vi "Import Groups.vi"(8 "error in (no error)":errorcluster, 10 "Path":path, 11 "BluelinesRedlines in":refnum<class "BluelinesRedlines.lvclass">) -> (0 "error out":errorcluster, 3 "BluelinesRedlines out":refnum<class "BluelinesRedlines.lvclass">)   [LabVIEW 2023, in "VolatusGUIElements.lvlib" / "BluelinesRedlines.lvclass"]
uses:
  BluelinesRedlines.lvclass
  VolatusGUI/BluelinesRedlines Source/BLRL Type.ctl
  BluelinesRedlines.lvclass/BluelinesRedlines.ctl
  User BluelinesRedlines/User BluelinesRedlines.lvclass
  VolatusErrorUtilities/MultiErrors/MultiErrors.lvclass/MultiErrors.ctl
  lv-cdm/CDM-Config/Config-JSON/Config-JSON.lvclass
  lv-cdm/CDM-Config/Config Storage/Config Storage.lvclass
  lv-cdm/CDM-Config/Config Manager/Config Manager.lvclass
  lv-cdm/CDM-Config/Config Element/Config Element.lvclass
  VolatusGUI/BluelinesRedlines Source/BluelinesRedlines Source.lvclass
  VolatusErrorUtilities/MultiErrors/MultiErrors.lvclass
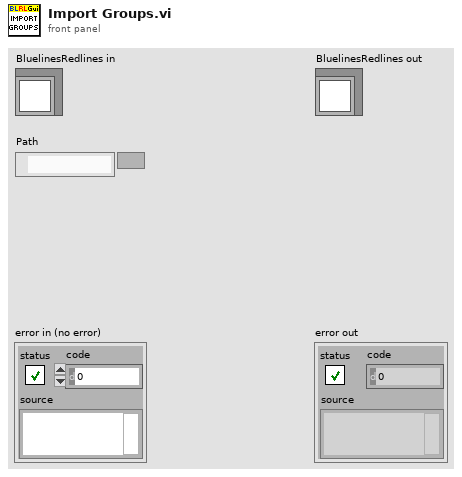
[diagram p1: front panel]
types:
  T1 = typedef "VolatusGUI.lvlib/BluelinesRedlines Source.lvclass/BLRL Type.ctl" = enum16{"Blueline", "Redline"}
  T2 = map{string, refnum<class "BluelinesRedlines Source.lvclass">}
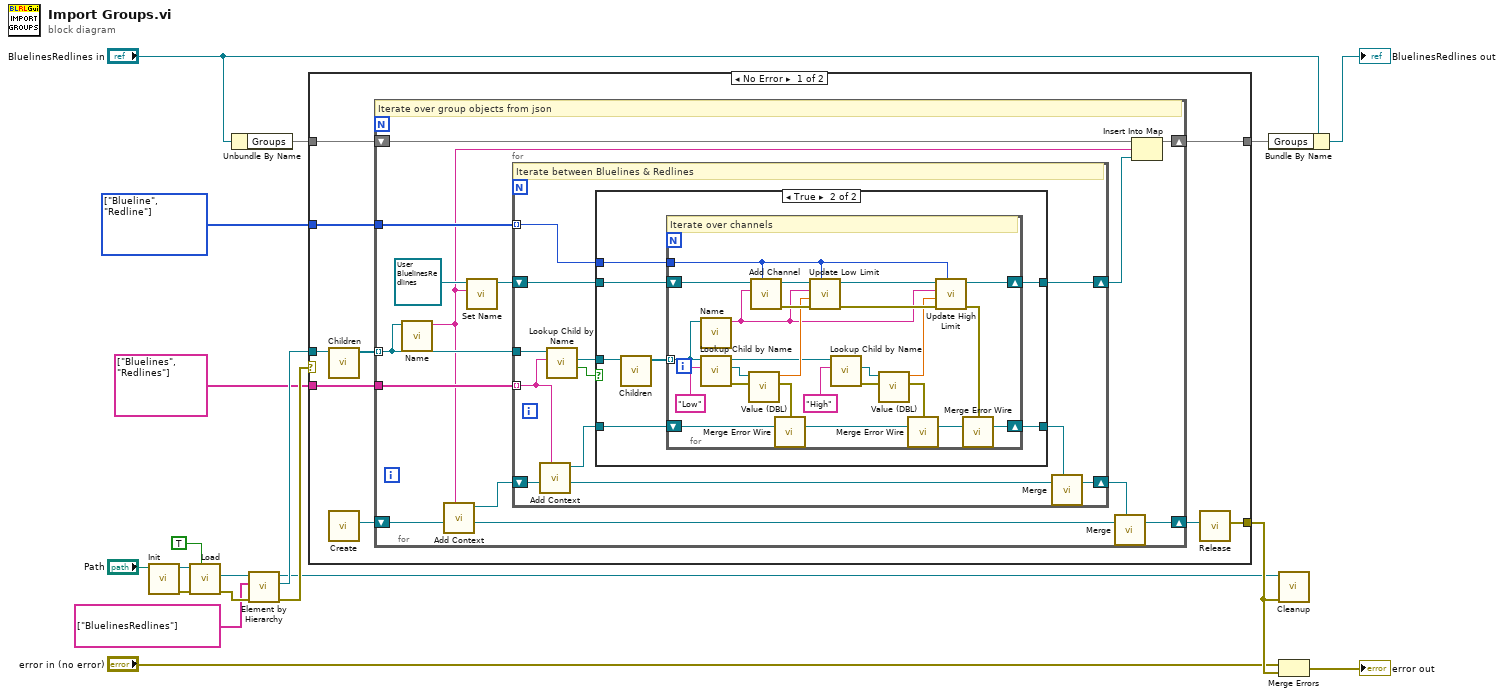
[diagram p0: block diagram]
diagram:
  w2 = T1[] [enum."Blueline", enum."Redline"] items=["Blueline", "Redline"]
  n1 = call "Init.vi"("Path"="Path") -> ("error out"=w15:errorcluster, "Config-JSON out"=w16:refnum<class "Config-JSON.lvclass">)  [unwired: 9 in]
  n2 = call "Load.vi"("Mutable (F)"=TRUE, "error in (no error)"=w15, "Config Storage in"=w16) -> ("error out"=w13:errorcluster, "Config"=w14:refnum<class "Config Manager.lvclass">)  [unwired: 6 in, 1 out]
  n3 = Unbundle By Name("BluelinesRedlines in") -> ("Groups"=w6:T2)
  n4 = call "Element by Hierarchy.vi"("error in (no error)"=w13, "Hierarchy"=string[] ["BluelinesRedlines"], "Config Manager in"=w14) -> ("error out"=w11:errorcluster, "Config Element"=w10:refnum<class "Config Element.lvclass">, "Config Manager out"=w8:refnum<class "Config Manager.lvclass">)  [unwired: 6 in]
  n5 = case shown="No Error" w11 {
    selector: w11 -> [_ w90]
    tunnel: w10 -> [w28 _]
    tunnel: [w21 w90] -> w19
    tunnel: w6 -> [w26 w89]
    tunnel: [w20 w89] -> w4
    tunnel: string[] ["Bluelines", "Redlines"] -> [w25 _]
    tunnel: w2 -> [w24 _]
    frame No Error {
      n6 = call "Children.vi"("Config Element in"=w28) -> ("Elements"=w27:refnum<class "Config Element.lvclass">[])  [unwired: 9 in, 1 out]
      n7 = call "Create.vi"() -> ("MultiErrors out"=w23:refnum<class "MultiErrors.lvclass">)  [unwired: 11 in]
      n8 = for {
        tunnel: w27 -> [w40] mode=indexing
        shift-right: [w36] -> w20
        shift-left: w26 -> [w37]
        tunnel: w25 -> [w39]
        tunnel: w24 -> [w38]
        shift-right: [w29] -> w22
        shift-left: w23 -> [w34]
        # "Iterate over group objects from json"
        n9 = call "Name.vi"("Config Element in"=w40) -> ("Name"=w33:string)  [unwired: 9 in, 1 out]
        n10 = call "Add Context.vi"("Context"=w33, "MultiErrors in"=w34) -> ("Original Context"=w31:refnum<class "MultiErrors.lvclass">, "Added Context"=w32:refnum<class "MultiErrors.lvclass">)  [unwired: 8 in]
        n11 = call "Set Name.vi"("Name"=w33, "User BluelinesRedlines in"=refnum<class "User BluelinesRedlines.lvclass"> refnum) -> ("User BluelinesRedlines out"=w41:refnum<class "User BluelinesRedlines.lvclass">)  [unwired: 8 in, 1 out]
        n12 = for {
          shift-right: [w49] -> w35
          shift-left: w41 -> [w50]
          tunnel: w40 -> [w54]
          tunnel: w39 -> [w47] mode=indexing
          tunnel: w38 -> [w53] mode=indexing
          shift-right: [w43] -> w30
          shift-left: w32 -> [w48]
          # "Iterate between Bluelines & Redlines"
          n13 = call "Add Context.vi"("Context"=w47, "MultiErrors in"=w48) -> ("Original Context"=w45:refnum<class "MultiErrors.lvclass">, "Added Context"=w46:refnum<class "MultiErrors.lvclass">)  [unwired: 8 in]
          n14 = call "Lookup Child by Name.vi"("Name"=w47, "Config Element in"=w54) -> ("Found"=w52:bool, "Child"=w51:refnum<class "Config Element.lvclass">)  [unwired: 6 in, 2 out]
          n15 = case shown="True" w52 {
            tunnel: w53 -> [_ w60]
            tunnel: w51 -> [_ w63]
            tunnel: w50 -> [w56 w61]
            tunnel: [w56 w59] -> w49
            tunnel: w46 -> [w55 w58]
            tunnel: [w55 w57] -> w44
            frame False {
            }
            frame True {
              n16 = call "Children.vi"("Config Element in"=w63) -> ("Elements"=w62:refnum<class "Config Element.lvclass">[])  [unwired: 9 in, 1 out]
              n17 = for {
                tunnel: w62 -> [w85] mode=indexing
                shift-right: [w71] -> w59
                shift-left: w61 -> [w87]
                tunnel: w60 -> [w75]
                shift-right: [w64] -> w57
                shift-left: w58 -> [w70]
                # "Iterate over channels"
                n18 = call "Name.vi"("Config Element in"=w85) -> ("Name"=w73:string)  [unwired: 9 in, 1 out]
                n19 = call "Lookup Child by Name.vi"("Name"="Low", "Config Element in"=w85) -> ("error out"=w84:errorcluster, "Child"=w83:refnum<class "Config Element.lvclass">, "Config Element out"=w77:refnum<class "Config Element.lvclass">)  [unwired: 6 in, 1 out]
                n20 = call "Value (DBL).vi"("error in (no error)"=w84, "Config Element in"=w83) -> ("error out"=w69:errorcluster, "DBL Value"=w82:dbl)  [unwired: 8 in]
                n21 = call "Add Channel.vi"("Type"=w75, "Channel Name"=w73, "User BluelinesRedlines in"=w87) -> ("error out"=w88:errorcluster, "User BluelinesRedlines out"=w86:refnum<class "User BluelinesRedlines.lvclass">)  [unwired: 7 in]
                n22 = call "Merge Error Wire.vi"("error in (no error)"=w69, "MultiErrors in"=w70) -> ("MultiErrors out"=w68:refnum<class "MultiErrors.lvclass">)  [unwired: 13 in]
                n23 = call "Update Low Limit.vi"("Type"=w75, "error in (no error)"=w88, "Low Limit"=w82, "Channel Name"=w73, "User BluelinesRedlines in"=w86) -> ("error out"=w74:errorcluster, "User BluelinesRedlines out"=w76:refnum<class "User BluelinesRedlines.lvclass">)  [unwired: 5 in]
                n24 = call "Lookup Child by Name.vi"("Name"="High", "Config Element in"=w77) -> ("error out"=w78:errorcluster, "Child"=w79:refnum<class "Config Element.lvclass">)  [unwired: 6 in, 2 out]
                n25 = call "Value (DBL).vi"("error in (no error)"=w78, "Config Element in"=w79) -> ("error out"=w67:errorcluster, "DBL Value"=w72:dbl)  [unwired: 8 in]
                n26 = call "Merge Error Wire.vi"("error in (no error)"=w67, "MultiErrors in"=w68) -> ("MultiErrors out"=w66:refnum<class "MultiErrors.lvclass">)  [unwired: 13 in]
                n27 = call "Update High Limit.vi"("Type"=w75, "error in (no error)"=w74, "High Limit"=w72, "Channel Name"=w73, "User BluelinesRedlines in"=w76) -> ("error out"=w65:errorcluster, "User BluelinesRedlines out"=w71:refnum<class "User BluelinesRedlines.lvclass">)  [unwired: 5 in]
                n28 = call "Merge Error Wire.vi"("error in (no error)"=w65, "MultiErrors in"=w66) -> ("MultiErrors out"=w64:refnum<class "MultiErrors.lvclass">)  [unwired: 13 in]
              }
            }
          }
          n29 = call "Merge.vi"("First Error In"=w45, "Second Error In"=w44) -> ("MultiErrors out"=w43:refnum<class "MultiErrors.lvclass">)  [unwired: 5 in]
        }
        n30 = call "Merge.vi"("First Error In"=w31, "Second Error In"=w30) -> ("MultiErrors out"=w29:refnum<class "MultiErrors.lvclass">)  [unwired: 5 in]
        n31 = Insert Into Map(map in=w37, key=w33, value=w35) -> (map out=w36:T2)  [unwired: 2 out]
      }
      n32 = call "Release.vi"("MultiErrors in"=w22) -> ("error out"=w21:errorcluster)  [unwired: 10 in]
    }
    frame Error {
    }
  }
  n33 = Bundle By Name(cluster="BluelinesRedlines in", "Groups"=w4) -> (→"BluelinesRedlines out":refnum<class "BluelinesRedlines.lvclass">)
  n34 = call "Cleanup.vi"("error in (no error)"=w19, "Config Manager in"=w8) -> ()  [unwired: 9 in, 1 out]
  n35 = Merge Errors("error in (no error)", w19) -> (→"error out":errorcluster)
